vi "Actor SD.vi"(4 "Creator Attributes":refnum<class "Attributes.lvclass">, 6 "Queue of Self Attributes":refnum<queue>, 7 "Alias":string, 9 "Queue of Error":refnum<queue>, 10 "Actor in":refnum<class "Actor.lvclass">) -> (0 "Error out":errorcluster, 2 "Actor out":refnum<class "Actor.lvclass">)   [LabVIEW 2020, in "jettl.lvlib" / "Actor.lvlib"]
uses:
  Actor.lvlib
  Attributes/Attributes/Attributes.lvclass
  Actor/Actor.lvclass
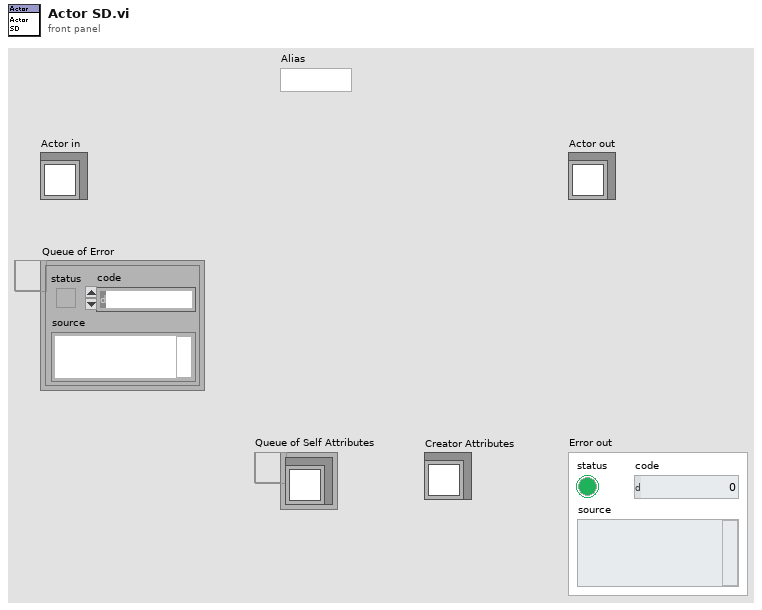
[diagram p1: front panel]
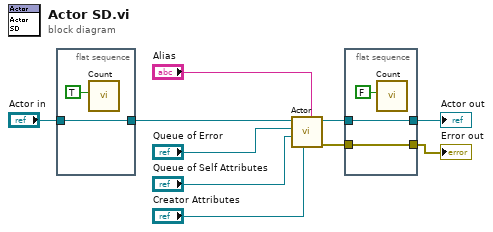
[diagram p0: block diagram]
diagram:
  n1 = flat-sequence {
    tunnel: [w11] -> w3
    tunnel: "Actor in" -> [w11]
    frame #0 {
      n2 = call "Count.vi"("Increment?"=TRUE) -> ()  [unwired: 11 in]
    }
  }
  n3 = call-dynamic "Actor.vi"("Alias"="Alias", "Creator Attributes"="Creator Attributes", "Queue of Self Attributes"="Queue of Self Attributes", "Queue of Error"="Queue of Error", "Actor in"=w3) -> ("Error out"=w8:errorcluster, "Actor out"=w9:refnum<class "Actor.lvclass">)  [unwired: 5 in]
  n4 = flat-sequence {
    tunnel: [w14] -> w10
    tunnel: w8 -> [w14]
    tunnel: [w13] -> w2
    tunnel: w9 -> [w13]
    frame #0 {
      n5 = call "Count.vi"("Increment?"=FALSE) -> ()  [unwired: 11 in]
    }
  }
  "Error out" <- w10
  "Actor out" <- w2
